vi "Properties Table.vi"(5 "Properties":T1=4211904 items=["SENSOR MODE"=4212128, "CCD MODE"=4212384, "READOUT MODE"=4211872, "ACTIVE VIEW INDEX"=4343136, "BITS PER CHANNEL"=4342976, "IMAGE PIXEL TYPE"=4343296, "BINNING"=4215968, "EXPOSURE TIME"=2049184, "CONTRAST GAIN"=3163312, "CONTRAST OFFSET"=3163328, "LIGHT MODE"=2114720, "SENSITIVITY"=2114992, "PHOTON IMAGING MODE"=2115200, "HIGH DYNAMIC RANGE MODE"=3163360, "WHITE BALANCE"=3163568, "TEMPERATURE"=2115232, "TEMPERATURE TARGET"=2115264, "SENSOR COOLER FAN"=2115296, "LINEBUNDLE HEIGHT"=4212192, "MECHANICAL SHUTTER"=2115488, "BACK FOCUS POSITION"=8422304, "TRIGGER CONNECTOR"=1066432, "TRIGGER SOURCE"=1066144, "OUTPUT TRIGGER SOURCE"=1852576, "TRIGGER GLOBAL EXPOSURE"=2049680, "FIRST TRIGGER BEHAVIOR"=2049696, "CHANNEL SYNC"=1852352, "READOUT DIRECTION"=4211904, "PRE HSYNC COUNT"=1852704, "INTERNAL LINE SPEED"=4191408, "INTERNAL LINE INVERVAL"=4191424], 8 "Handle In":u32) -> (0 "Values Out":dbl[](array[numeric]), 1 "Value Stirngs Out":string[](array[string]), 2 "Row Headers":string[](array[string]), 3 "Handle Out":u32)   [LabVIEW 2015]
uses:
  Camera Properties.ctl
panel:
  in  "Cluster":cluster{"String":string, "Combo Box":string}
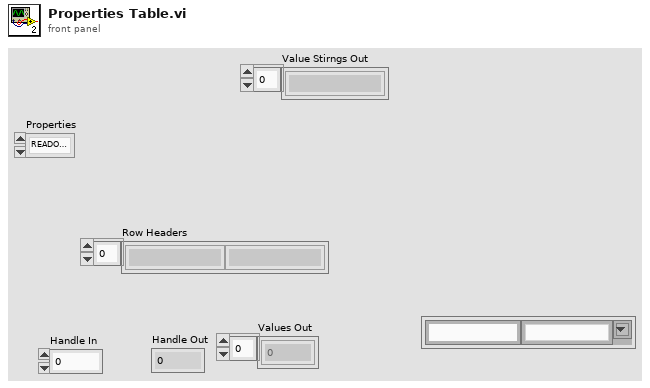
[diagram p1: front panel]
types:
  T1 = typedef "Camera Properties.ctl" = u32
  T2 = typedef "LVStringsAndValuesArrayTypeDef_U32.ctl" = cluster{"String":string, "Value":u32}[]
  T3 = cluster{"Cluster":cluster{"String":string, "Combo Box":string}, "Cluster":cluster{"String":string, "Combo Box":string}}
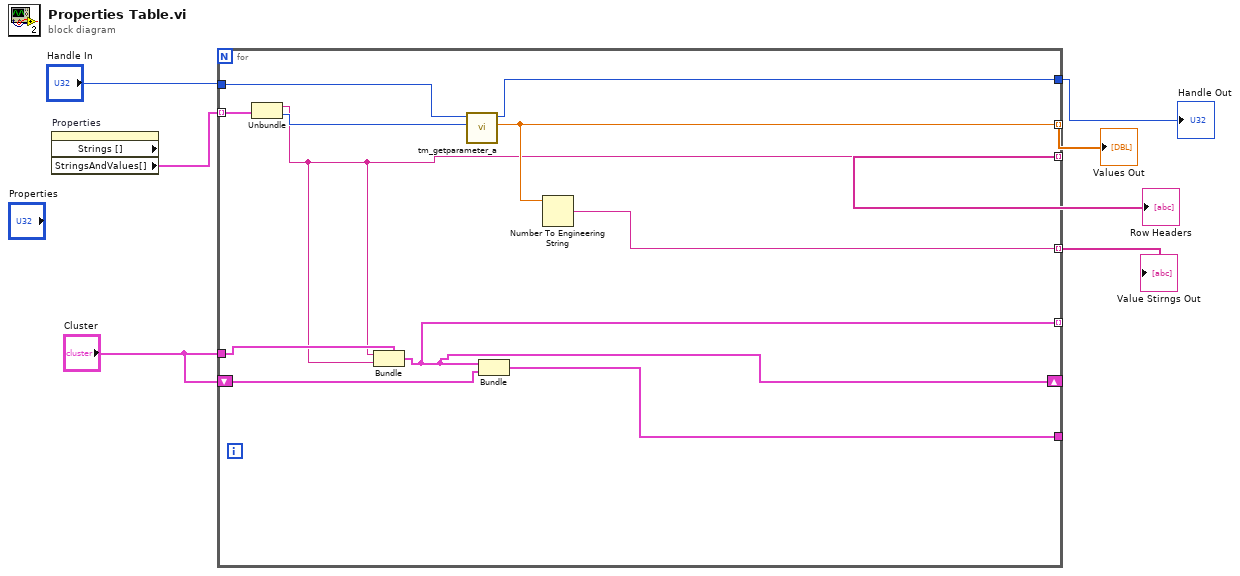
[diagram p0: block diagram]
diagram:
  n1 = property on="Properties" class="Ring (strict)" props=["Strings []", "StringsAndValues[]"]() -> ("StringsAndValues[]"=w2:T2)  [unwired: 2 in, 3 out]
  n2 = for {
    tunnel: w2 -> [w16] mode=indexing
    tunnel: "Handle In" -> [w18]
    tunnel: [w17] -> w6
    tunnel: [w9] -> w5 mode=indexing
    tunnel: [w15] -> w4 mode=indexing
    tunnel: [w14] -> w3 mode=indexing
    tunnel: "Cluster" -> [w11]
    shift-right: [w8] -> _
    shift-left: "Cluster" -> [w12]
    tunnel: [w10] -> _
    tunnel: [w8] -> _ mode=indexing
    n3 = Unbundle(w16) -> ("String"=w9:string, "Value"=w13:u32)
    n4 = Bundle(cluster=w11, "String"=w9, "Combo Box"=w9) -> (w8:cluster{"String":string, "Combo Box":string})
    n5 = call "tm_getparameter_a.vi"("Parameter"=w13, "Handle in"=w18) -> ("Value out"=w15:dbl, "Handle out"=w17:u32)  [unwired: 7 in, 1 out]
    n6 = Bundle("Cluster"=w8, "Cluster"=w12) -> (w10:T3)  [unwired: 1 in]
    n7 = Number To Engineering String(4:w15) -> (0:w14:string)  [unwired: 3 in]
  }
  "Handle Out" <- w6
  "Row Headers" <- w5
  "Values Out" <- w4
  "Value Stirngs Out" <- w3
